vi "get device usb strings.vi"(8 "error in (no error)":errorcluster, 11 "Device Index":u32) -> (0 "error out":errorcluster, 2 "function return":i32, 3 "Device USB Strings":T1)   [LabVIEW 2015, in "rtlsdr.lvlib"]
doc: "Retrieves manufacturer, product, and serial number from the device specified by index."
uses:
  rtlsdr.lvlib
  rtlsdr/rtlsdr.dll
panel:
  in  "serial":string
  in  "product":string
  in  "manufact":string
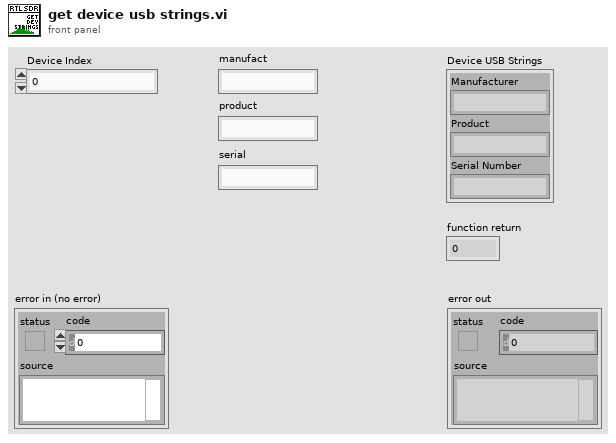
[diagram p1: front panel]
types:
  T1 = cluster{"Manufacturer":string, "Product":string, "Serial Number":string}
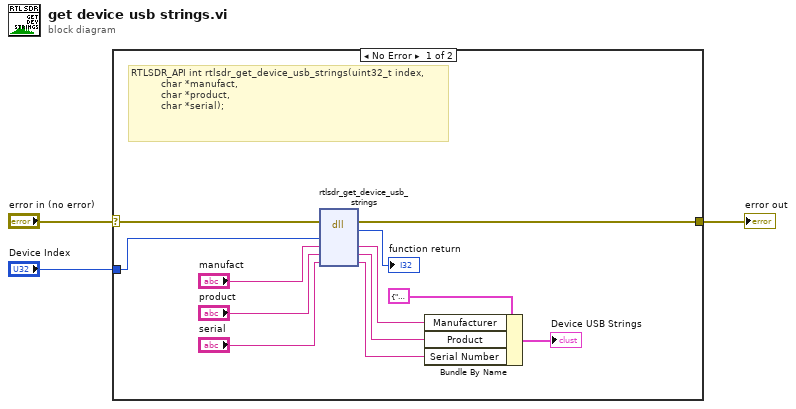
[diagram p0: block diagram]
diagram:
  n1 = case shown="No Error" "error in (no error)" {
    selector: "error in (no error)" -> [w5 w16]
    tunnel: "Device Index" -> [w4 _]
    tunnel: [w11 w16] -> w2
    frame No Error {
      # "RTLSDR_API int rtlsdr_get_device_usb_strings(uint32_t index,\n\t\t\t\t\t     char *manufact,\n\t\t\t\t\t     char *product,\n\t\t\t\t\t     char *serial);"
      n2 = dll-call lib="C:/Users/TheDoctor/Documents/Projects/Labview Libraries/rtlsdr/rtlsdr.*" fn="rtlsdr_get_device_usb_strings"(error in=w5, "index"=w4, "manufact"="manufact", "product"="product", "serial"="serial") -> (error out=w11:errorcluster, "return type"=→"function return":i32, "manufact"=w9:string, "product"=w8:string, "serial"=w7:string)  [unwired: 3 in, 1 out]
      n3 = Bundle By Name(cluster=T1 {"Manufacturer"="", "Product"="", "Serial Number"=""}, "Manufacturer"=w9, "Product"=w8, "Serial Number"=w7) -> (→"Device USB Strings":T1)
    }
    frame Error {
    }
  }
  "error out" <- w2
